vi "LVClass_ClosedLoopSmoothing_Ctor.vi"(0 "ClosedLoopSmoothing in":refnum<class "ClosedLoopSmoothing.lvclass">, 5 "CLoopSmoothingParams":T1, 11 "error in (no error)":errorcluster) -> (4 "ClosedLoopSmoothing out":refnum<class "ClosedLoopSmoothing.lvclass">, 15 "error out":errorcluster)   [LabVIEW 2020, in "ClosedLoopSmoothing.lvclass"]
uses:
  ClosedLoopSmoothing.lvclass
  ClosedLoopSmoothingParameters.ctl
  Handle creation.ctl
  ClosedLoopSmoothing.lvclass/ClosedLoopSmoothing.ctl
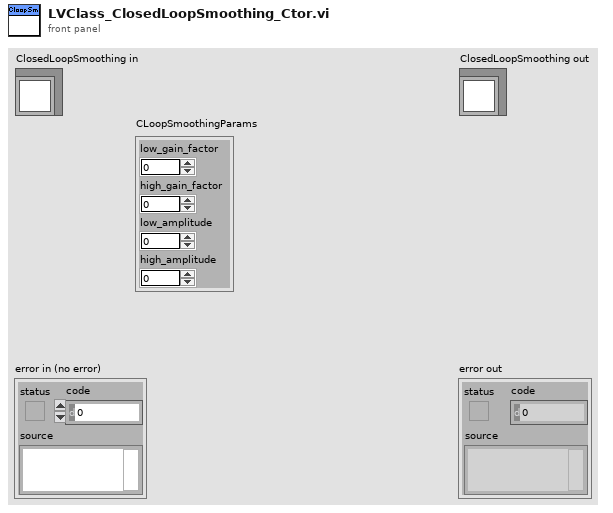
[diagram p1: front panel]
types:
  T1 = typedef "ClosedLoopSmoothingParameters.ctl" = cluster{"low_gain_factor":sgl, "high_gain_factor":sgl, "low_amplitude":i32, "high_amplitude":i32}
  T2 = typedef "Handle creation.ctl" = enum16{"By ctor", "By write function"}
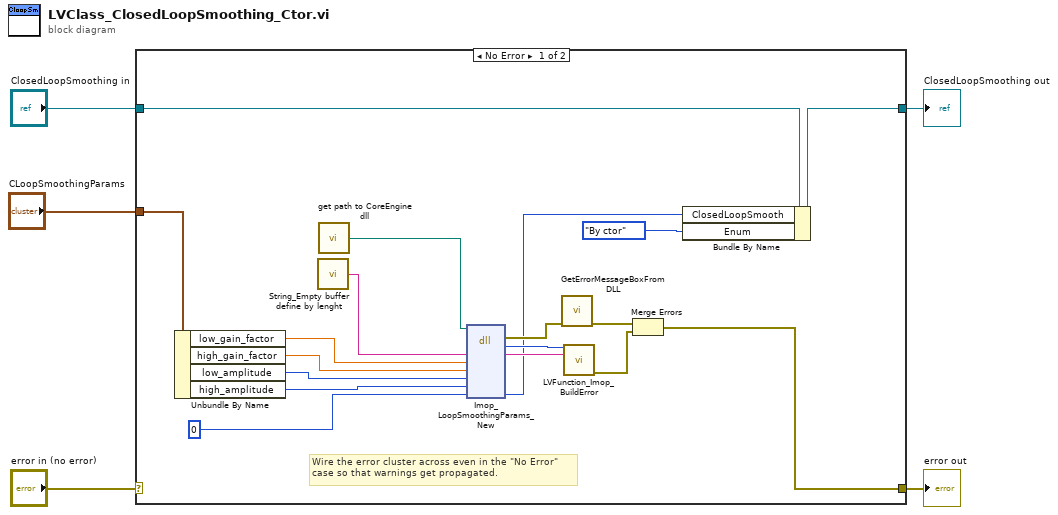
[diagram p0: block diagram]
diagram:
  n1 = case shown="No Error" "error in (no error)" {
    selector: "error in (no error)" -> [_ w25]
    tunnel: [w11 w25] -> w4
    tunnel: [w12 w24] -> w2
    tunnel: "ClosedLoopSmoothing in" -> [w13 w24]
    tunnel: "CLoopSmoothingParams" -> [w10 _]
    frame No Error {
      # "Wire the error cluster across even in the \"No Error\"\ncase so that warnings get propagated."
      n2 = Unbundle By Name(w10) -> ("low_gain_factor"=w9:sgl, "high_gain_factor"=w8:sgl, "low_amplitude"=w7:i32, "high_amplitude"=w6:i32)
      n3 = call "String_Empty buffer define by lenght.vi"() -> ("Empty buffer"=w23:string)  [unwired: 1 in]
      n4 = call "get path to CoreEngine dll.vi"() -> ("path to c_interface_vc100.dll"=w14:path)  [unwired: 12 in, 3 out]
      n5 = dll-call lib="D:/soft/HASO_v3/SVN_trunk/ImOpCoreEngine4_LV2011/DLLs/c_interface_vc100.dll" fn="Imop_LoopSmoothingParams_New"(path in=w14, "message"=w23, "low_gain_factor"=w9, "high_gain_factor"=w8, "low_amplitude"=w7, "High_amplitude"=w6, "WavefrontCorrectorSet"=0 ("Pupil")) -> (error out=w20:errorcluster, "return type"=w21:i32, "message"=w22:string, "WavefrontCorrectorSet"=w18:i32)  [unwired: 6 in, 1 out]
      n6 = call "GetErrorMessageBoxFromDLL.vi"("error IN"=w20) -> ("error OUT"=w16:errorcluster)  [unwired: 10 in]
      n7 = call "LVFunction_Imop_BuildError.vi"("code"=w21, "String to Prepend to source (\"\")"=w22) -> ("error out"=w15:errorcluster)  [unwired: 13 in]
      n8 = Merge Errors(w16, w15) -> (w11:errorcluster)
      n9 = Bundle By Name(cluster=w13, "ClosedLoopSmooth"=w18, "Enum"=Handle_creation."By ctor" ("Pupil ptr create")) -> (w12:refnum<class "ClosedLoopSmoothing.lvclass">)
    }
    frame Error {
    }
  }
  "error out" <- w4
  "ClosedLoopSmoothing out" <- w2
